vi "GetESD.vi"(8 "error in (no error)":errorcluster caption="错误输入（无错误）", 10 "Addr":u8, 11 "DevControl 输入":refnum<class "DevControl.lvclass"> caption="DNL_LabVIEW Object in") -> (0 "error out":errorcluster caption="错误输出", 1 "ÑbÖÃ î‘B":T1, 3 "DevControl 输出":refnum<class "DevControl.lvclass"> caption="DNL_LabVIEW Object out")   [LabVIEW 2012, in "DevControl.lvclass"]
uses:
  DevControl.lvclass
  SupportVi/DevState.ctl
  SupportVi/DevCmd.ctl
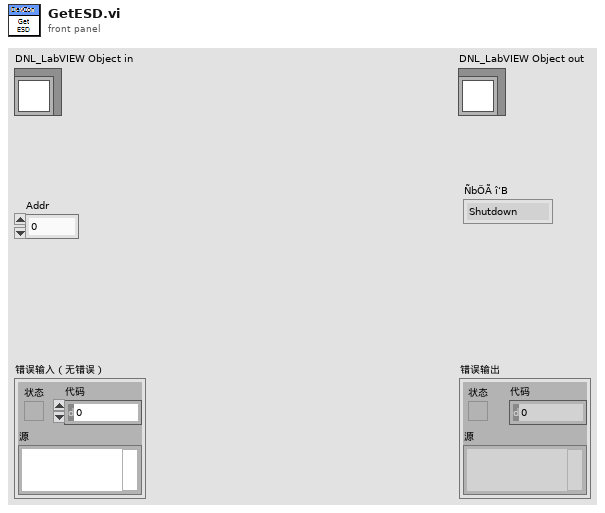
[diagram p1: front panel]
types:
  T1 = typedef "DevControl.lvclass/DevState.ctl" = enum16{"Shutdown", "PASS", "FAIL", "Idle", "Noresponse"}
  T2 = typedef "DevControl.lvclass/DevCmd.ctl" = u8
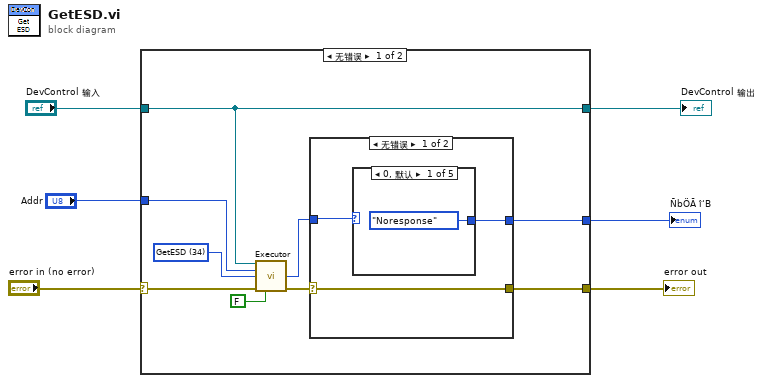
[diagram p0: block diagram]
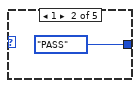
[diagram p2: hidden frame]
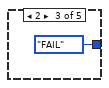
[diagram p3: hidden frame]
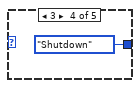
[diagram p4: hidden frame]
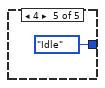
[diagram p5: hidden frame]
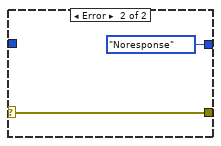
[diagram p6: hidden frame]
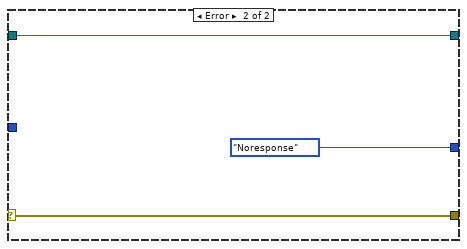
[diagram p7: hidden frame]
diagram:
  n1 = case shown="无错误" "error in (no error)" {
    selector: "error in (no error)" -> [w12 w28]
    tunnel: [w8 w28] -> w5
    tunnel: [w15 w27] -> w3
    tunnel: "DevControl 输入" -> [w15 w27]
    tunnel: "Addr" -> [w14 _]
    tunnel: [w9 DevState."Noresponse" ("ÑbÖÃ î‘B")] -> w1
    frame No Error {
      w13 = T2 34 items=["WriteAddr"=81, "Enable"=80, "Red"=66, "Green"=65, "TurnOn"=49, "Shutdown"=48, "GetESD"=34] ("DevCmd")
      n2 = call-dynamic "Executor.vi"("DevControl 输入"=w15, "Addr"=w14, "DevCmd"=w13, "error in (no error)"=w12, "ChkDat?"=FALSE) -> ("Data"=w10:u8, "error out"=w11:errorcluster)  [unwired: 8 in, 1 out]
      n3 = case shown="无错误" w11 {
        selector: w11 -> [w16 w24]
        tunnel: w10 -> [w18 _]
        tunnel: [w17 DevState."Noresponse" ("ÑbÖÃ î‘B")] -> w9
        tunnel: [w16 w24] -> w8
        frame No Error {
          n4 = case shown="0, 默认" w18 {
            tunnel: [DevState."Noresponse" ("ÑbÖÃ î‘B") DevState."PASS" ("ÑbÖÃ î‘B") DevState."FAIL" ("ÑbÖÃ î‘B") DevState."Shutdown" ("ÑbÖÃ î‘B") DevState."Idle" ("ÑbÖÃ î‘B")] -> w17
            frame 0, Default {
            }
            frame 1 {
            }
            frame 2 {
            }
            frame 3 {
            }
            frame 4 {
            }
          }
        }
        frame Error {
        }
      }
    }
    frame Error {
    }
  }
  "error out" <- w5
  "DevControl 输出" <- w3
  "ÑbÖÃ î‘B" <- w1
